vi "Create System Image.vi"   [LabVIEW 2017, in "nisyscfg.lvlib"]
doc: "Creates a system image file or folder—a copy of the file contents on a primary hard drive of a system. You may want to create a system image to restore a system to its original state or to deploy the image to other systems."
uses:
  <vilib>/nisyscfg/nisyscfg.lvlib
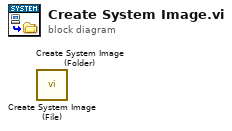
[diagram p0: block diagram]
diagram:
  n1 = call <vilib>:"Create System Image (File).vi"() -> ()  [unwired: 9 in, 3 out]
  n2 = call <vilib>:"Create System Image (Folder).vi"() -> ()  [unwired: 9 in, 3 out]
